vi "Flywheel_Simulated_Hardware.vi"() -> ()   [LabVIEW 2019]
panel:
  out "measured flywheel_velocity(rot/s)":dbl
  out "true_flywheel_position":dbl
  in  "Friction":dbl
  in  "Flywheel_Mass(kg)":dbl
  in  "a_init":dbl
  in  "v_init":dbl
  in  "x_init":dbl
  out "flywheel_acceleration":dbl
  out "true_flywheel_velocity":dbl
  out "measured flywheel_position(rot)":dbl
  in  "Flywheel_Power(u)":dbl
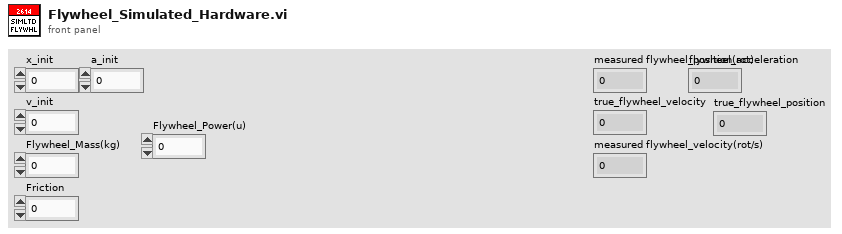
[diagram p1: front panel]
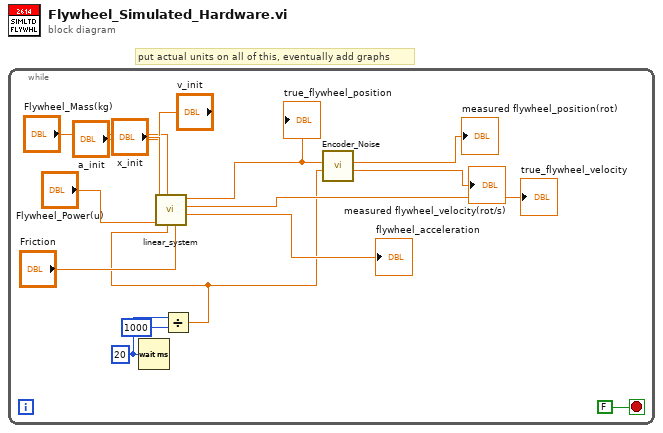
[diagram p0: block diagram]
diagram:
  # "put actual units on all of this, eventually add graphs"
  n1 = while {
    stop <- FALSE stop-if-true
    w4 = u32 20 ("milliseconds to wait")
    n2 = Wait (ms)(milliseconds to wait=w4) -> ()  [unwired: 1 out]
    n3 = Divide(x=w4, y=u32 1000) -> (x/y=w2:dbl)
    n4 = call "linear_system.vi"("c(friction)"="Friction", "delta_t"=w2, "m(mass)"="Flywheel_Mass(kg)", "u_in(input force)"="Flywheel_Power(u)", "a_init"="a_init", "v_init"="v_init", "x_init"="x_init") -> ("a_out"=→"flywheel_acceleration":dbl, "v_out"=→"true_flywheel_velocity":dbl, "x_out"=w6:dbl)  [unwired: 2 in]
    "true_flywheel_position" <- w6
    n5 = call "Encoder_Noise.vi"("dt(s)"=w2, "True Position(rotations)"=w6) -> ("Measured Velocity(rotations/sec)"=→"measured flywheel_velocity(rot/s)":dbl, "Measured Position(rotations)"=→"measured flywheel_position(rot)":dbl)  [unwired: 8 in]
  }
